vi "CS장난감용클라.vi"() -> ()   [LabVIEW 2018]
uses:
  <vilib>/LabVIEW Open Source Project/MQTT TCP Connection/MQTT_TCP/Connection/TCPConnection.lvclass
  C:/Program Files (x86)/National Instruments/LabVIEW 2018/vi.lib/LabVIEW Open Source Project/Connection/Connection/Connection.lvclass
  <vilib>/LabVIEW Open Source Project/Connection/Connection/Connection.lvclass
panel:
  in  "파일(대화 상자 사용)":path
  in  "Folder Path":path caption="다운로드  경로"
  in  "다운로드":bool
  out "선택한 파일":string
  in  "리스트":i32(listbox)=-1
  in  "리스트 업데이트":bool
  out "정지 Echo":string
  in  "정지":bool
  out "Comm OK":bool
  out "server connected":bool
  in  "전송":bool
  in  "보낸 문자열":string
  out "받은 문자열":string
  out "client session error":errorcluster
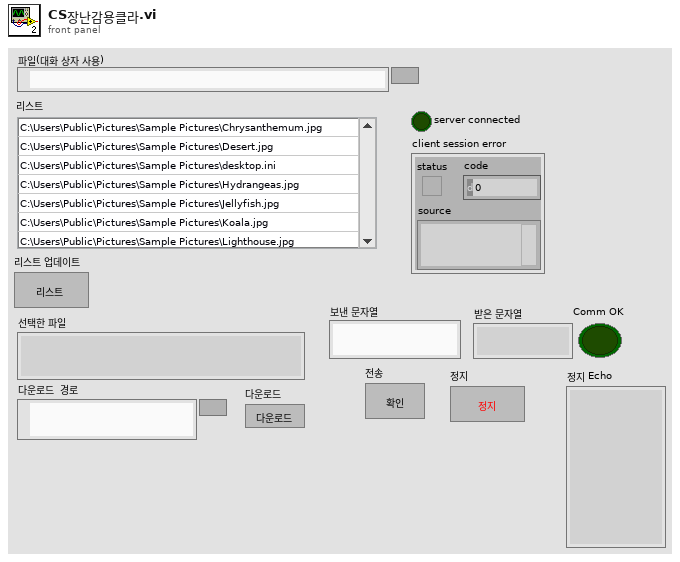
[diagram p1: front panel]
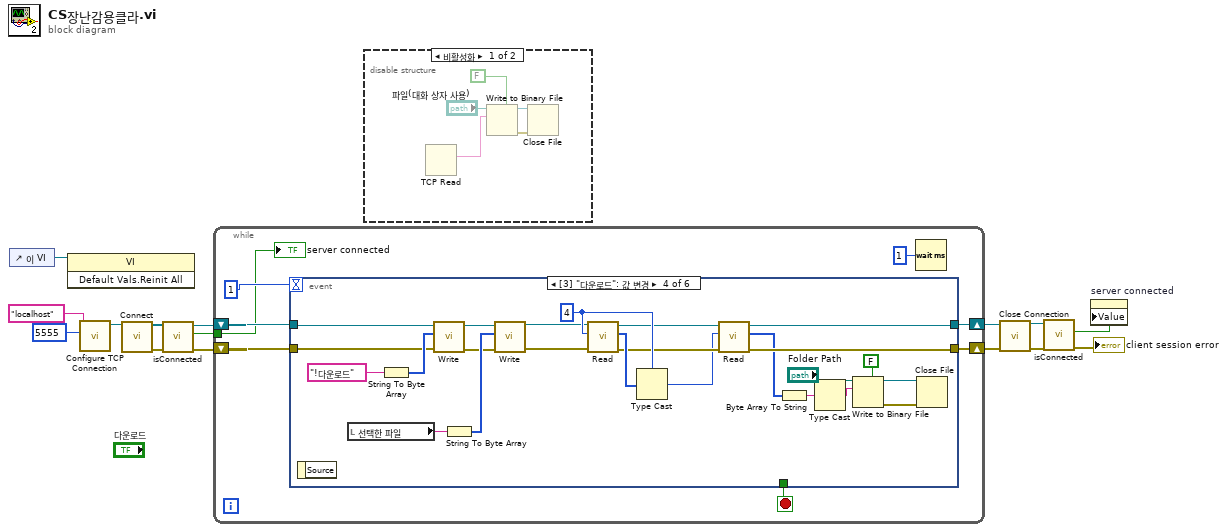
[diagram p0: block diagram]
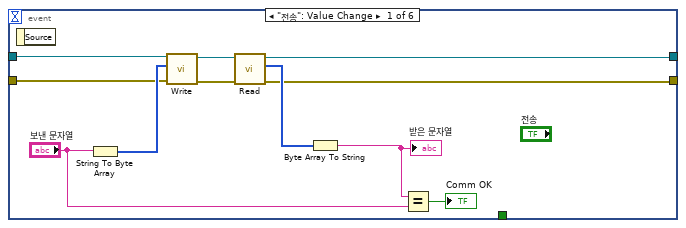
[diagram p3: hidden frame]
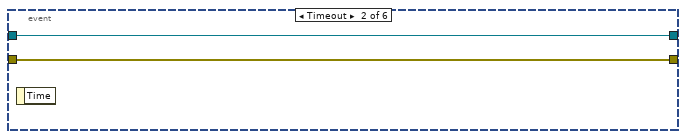
[diagram p4: hidden frame]
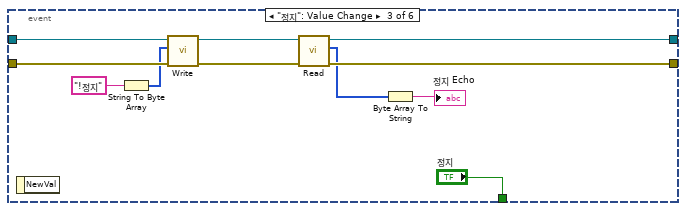
[diagram p5: hidden frame]
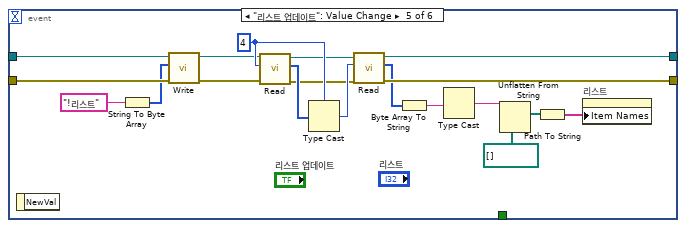
[diagram p6: hidden frame]
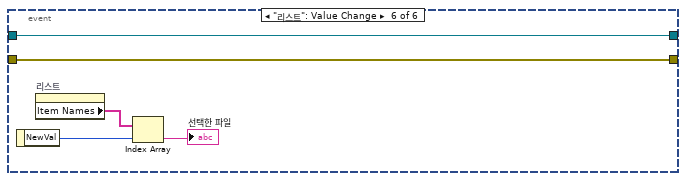
[diagram p7: hidden frame]
diagram:
  n1 = control-ref of="이 VI"() -> (w5:refnum<vi>)
  n2 = invoke class="VI" method="Default Vals.Reinit All"(reference=w5) -> ()  [unwired: 2 in, 3 out]
  n3 = call <vilib>:"Configure TCP Connection.vi"("remote port (80)"=u16 5555, "address (localhost)"="localhost") -> ("TCPConnection"=w13:refnum<class "TCPConnection.lvclass">)  [unwired: 8 in, 1 out]
  n4 = call <vilib>:"Connect.vi"("Connection in"=w13) -> ("error out"=w9:errorcluster, "Connection out"=w7:refnum<class "TCPConnection.lvclass">)  [unwired: 9 in]
  n5 = call <vilib>:"isConnected.vi"("error in (no error)"=w9, "Connection in"=w7) -> ("error out"=w8:errorcluster, "connected"=w10:bool, "Connection out"=w6:refnum<class "TCPConnection.lvclass">)  [unwired: 7 in]
  n6 = while {
    tunnel: w10 -> [w16]
    shift-right: [w23] -> w15
    shift-left: w8 -> [w21]
    shift-right: [w22] -> w14
    shift-left: w6 -> [w20]
    stop <- w17 stop-if-true
    n7 = event shown="[3] \"다운로드\": 값 변경" {
      selector: _ -> [_ _ _ _ _ _]
      dyn-events: _ -> [_ _ _ _ _ _]
      timeout: 1 -> [_ _ _ _ _ _]
      tunnel: [w30 w35 w41 w54 w86 w92] -> w23
      tunnel: [w29 w36 w42 w55 w87 w91] -> w22
      tunnel: w21 -> [w27 w35 w46 w65 w89 w92]
      tunnel: w20 -> [w26 w36 w47 w66 w90 w91]
      tunnel: [_ _ "정지" _ _ _] -> w17
      event "전송": Value Change {
        n8 = event-data() -> ()  [unwired: 1 in, 1 out]
        n9 = String To Byte Array(string="보낸 문자열") -> (unsigned byte array=w32:u8[])
        n10 = call <vilib>:"Write.vi"("error in (no error)"=w27, "Bytes"=w32, "Connection in"=w26) -> ("error out"=w33:errorcluster, "Connection"=w34:refnum<class "TCPConnection.lvclass">)  [unwired: 7 in]
        n11 = call <vilib>:"Read.vi"("error in (no error)"=w33, "TCPConnection in"=w34) -> ("error out"=w30:errorcluster, "Bytes"=w31:u8[], "TCPConnection out"=w29:refnum<class "TCPConnection.lvclass">)  [unwired: 5 in, 2 out]
        n12 = Byte Array To String(unsigned byte array=w31) -> (string=w24:string)
        "받은 문자열" <- w24
        n13 = Equal?(x=w24, y="보낸 문자열") -> (x = y?=→"Comm OK":bool)
      }
      event Timeout {
        n14 = event-data() -> ()  [unwired: 1 in, 1 out]
      }
      event "정지": Value Change {
        n15 = event-data() -> ()  [unwired: 1 in, 1 out]
        n16 = String To Byte Array(string="!정지" ("문자열")) -> (unsigned byte array=w39:u8[])
        n17 = call <vilib>:"Write.vi"("error in (no error)"=w46, "Bytes"=w39, "Connection in"=w47) -> ("error out"=w43:errorcluster, "Connection"=w44:refnum<class "TCPConnection.lvclass">)  [unwired: 7 in]
        n18 = call <vilib>:"Read.vi"("error in (no error)"=w43, "TCPConnection in"=w44) -> ("error out"=w41:errorcluster, "Bytes"=w38:u8[], "TCPConnection out"=w42:refnum<class "TCPConnection.lvclass">)  [unwired: 5 in, 2 out]
        n19 = Byte Array To String(unsigned byte array=w38) -> (string=→"정지 Echo":string)
      }
      event "다운로드": Value Change {
        w60 = 4 ("bytes to read (100)")
        n20 = event-data() -> ()  [unwired: 1 in, 1 out]
        n21 = local read "선택한 파일"() -> (w71:string)
        n22 = String To Byte Array(string="!다운로드" ("문자열")) -> (unsigned byte array=w67:u8[])
        n23 = call <vilib>:"Write.vi"("error in (no error)"=w65, "Bytes"=w67, "Connection in"=w66) -> ("error out"=w63:errorcluster, "Connection"=w64:refnum<class "TCPConnection.lvclass">)  [unwired: 7 in]
        n24 = String To Byte Array(string=w71) -> (unsigned byte array=w70:u8[])
        n25 = call <vilib>:"Write.vi"("error in (no error)"=w63, "Bytes"=w70, "Connection in"=w64) -> ("error out"=w56:errorcluster, "Connection"=w57:refnum<class "TCPConnection.lvclass">)  [unwired: 7 in]
        n26 = call <vilib>:"Read.vi"("error in (no error)"=w56, "bytes to read (100)"=w60, "TCPConnection in"=w57) -> ("error out"=w58:errorcluster, "Bytes"=w61:u8[], "TCPConnection out"=w59:refnum<class "TCPConnection.lvclass">)  [unwired: 4 in, 2 out]
        n27 = Type Cast(type=w60, x=w61) -> (*(type *) &x=w48:i32)
        n28 = call <vilib>:"Read.vi"("error in (no error)"=w58, "bytes to read (100)"=w48, "TCPConnection in"=w59) -> ("error out"=w54:errorcluster, "Bytes"=w51:u8[], "TCPConnection out"=w55:refnum<class "TCPConnection.lvclass">)  [unwired: 4 in, 2 out]
        n29 = Byte Array To String(unsigned byte array=w51) -> (string=w50:string)
        n30 = Type Cast(x=w50) -> (*(type *) &x=w49:string)  [unwired: 1 in]
        n31 = Write to Binary File(file (use dialog)="Folder Path", data=w49, 5:FALSE ("배열 또는 문자열 크기를 앞에 추가? (참)")) -> (refnum out=w68:refnum<file>, error out=w69:errorcluster)  [unwired: 3 in, 1 out]
        n32 = Close File(refnum=w68, error in=w69) -> ()  [unwired: 2 out]
      }
      event "리스트 업데이트": Value Change {
        w81 = 4 ("bytes to read (100)")
        n33 = event-data() -> ()  [unwired: 1 in, 1 out]
        n34 = String To Byte Array(string="!리스트" ("문자열")) -> (unsigned byte array=w85:u8[])
        n35 = call <vilib>:"Write.vi"("error in (no error)"=w89, "Bytes"=w85, "Connection in"=w90) -> ("error out"=w72:errorcluster, "Connection"=w73:refnum<class "TCPConnection.lvclass">)  [unwired: 7 in]
        n36 = call <vilib>:"Read.vi"("error in (no error)"=w72, "bytes to read (100)"=w81, "TCPConnection in"=w73) -> ("error out"=w78:errorcluster, "Bytes"=w82:u8[], "TCPConnection out"=w79:refnum<class "TCPConnection.lvclass">)  [unwired: 4 in, 2 out]
        n37 = Type Cast(type=w81, x=w82) -> (*(type *) &x=w80:i32)
        n38 = call <vilib>:"Read.vi"("error in (no error)"=w78, "bytes to read (100)"=w80, "TCPConnection in"=w79) -> ("error out"=w86:errorcluster, "Bytes"=w84:u8[], "TCPConnection out"=w87:refnum<class "TCPConnection.lvclass">)  [unwired: 4 in, 2 out]
        n39 = Byte Array To String(unsigned byte array=w84) -> (string=w77:string)
        n40 = Type Cast(x=w77) -> (*(type *) &x=w76:string)  [unwired: 1 in]
        n41 = Unflatten From String(type=path[] [], binary string=w76) -> (value=w74:path[])  [unwired: 3 in, 2 out]
        n42 = Path To String(path=w74) -> (string=w75:string[])
        n43 = property on="리스트" class="LstBox (엄격한)"("Item Names"=w75) -> ()  [unwired: 2 in, 2 out]
      }
      event "리스트": Value Change {
        n44 = event-data() -> ("NewVal"=w95:i32)  [unwired: 1 in]
        n45 = property on="리스트" class="LstBox (엄격한)"() -> ("Item Names"=w94:string[])  [unwired: 2 in, 2 out]
        n46 = Index Array(array=w94, index=w95) -> (element=→"선택한 파일":string)
      }
    }
    n47 = Wait (ms)(milliseconds to wait=u32 1 ("대기 시간 (ms)")) -> ()  [unwired: 1 out]
    "server connected" <- w16
  }
  n48 = disable-structure shown="비활성화" {
    frame Disabled {
      n49 = TCP Read() -> (data out=w98:string)  [unwired: 5 in, 2 out]
      n50 = Write to Binary File(file (use dialog)="파일(대화 상자 사용)", data=w98, 5:FALSE ("배열 또는 문자열 크기를 앞에 추가? (참)")) -> (refnum out=w96:refnum<file>, error out=w97:errorcluster)  [unwired: 3 in, 1 out]
      n51 = Close File(refnum=w96, error in=w97) -> ()  [unwired: 2 out]
    }
    frame Enabled {
    }
  }
  n52 = call <vilib>:"Close Connection.vi"("error in (no error)"=w15, "Connection in"=w14) -> ("error out"=w3:errorcluster, "No Connection"=w4:refnum<class "TCPConnection.lvclass">)  [unwired: 8 in]
  n53 = call <vilib>:"isConnected.vi"("error in (no error)"=w3, "Connection in"=w4) -> ("error out"=→"client session error":errorcluster, "connected"=w1:bool)  [unwired: 7 in, 1 out]
  n54 = property on="server connected" class="Bool (엄격한)"("Value"=w1) -> ()  [unwired: 2 in, 2 out]
